vi "FTW-Endpoint-Multipart-Receive.vi"(0 "FTW Endpoint":refnum<class "FTW-Endpoint-Notifier.lvclass">, 5 "Timeout":i32 format="%dmsec", 11 "error in":errorcluster) -> (4 "FTW Endpoint out":refnum<class "FTW-Endpoint-Notifier.lvclass">, 6 "Message Received":string[](array[string]), 8 "Timed out?":bool, 15 "error out":errorcluster)   [LabVIEW 2013, in "FTW-Actor.lvlib" / "FTW-Endpoint-Notifier.lvclass"]
uses:
  FTW-Endpoint-Notifier.lvclass
  FTW-Endpoint-Notifier.lvclass/FTW-Endpoint-Notifier.ctl
panel:
  # "Inputs"
  # "Outputs"
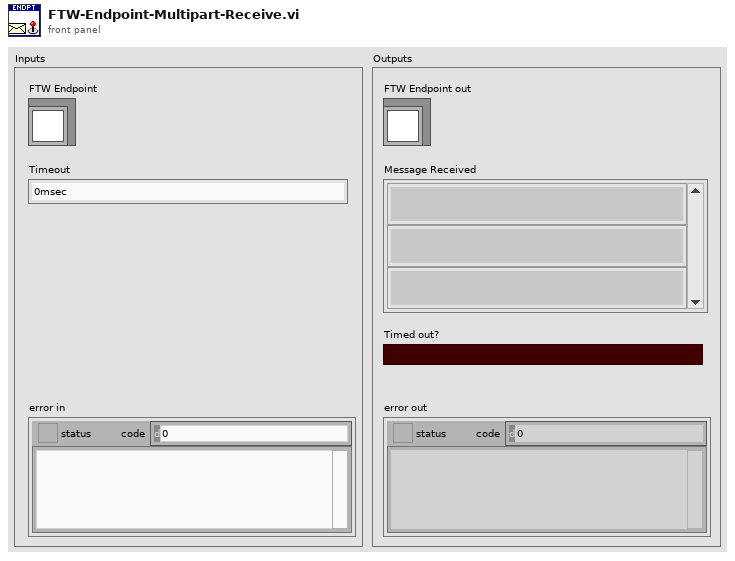
[diagram p1: front panel]
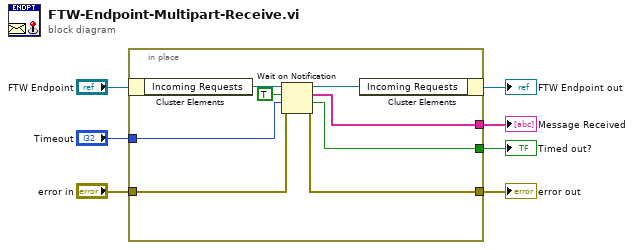
[diagram p0: block diagram]
diagram:
  n1 = in-place {
    in-place-border: [w12] -> w7
    in-place-border: "error in" -> [w13]
    in-place-border: "Timeout" -> [w14]
    in-place-border: [w10] -> w2
    in-place-border: [w9] -> w1
    n2 = in-place-cluster #1("FTW Endpoint") -> ("Incoming Requests"=w15:refnum<notifier>)
    n3 = Wait on Notification(notifier=w15, ignore previous (F)=TRUE, timeout in ms (-1)=w14, error in (no error)=w13) -> (notifier out=w11:refnum<notifier>, notification=w10:string[], timed out?=w9:bool, error out=w12:errorcluster)
    n4 = in-place-cluster #1("Incoming Requests"=w11) -> (→"FTW Endpoint out":refnum<class "FTW-Endpoint-Notifier.lvclass">)
  }
  "error out" <- w7
  "Message Received" <- w2
  "Timed out?" <- w1
